vi "highlightRows.vi"(8 "error in (no error)":errorcluster, 10 "Goal.lvclass":refnum<class "Goal.lvclass">, 11 "TransactionListUserInterface in":refnum<class "TransactionListUserInterface.lvclass">) -> (0 "error out":errorcluster, 3 "TransactionListUserInterface out":refnum<class "TransactionListUserInterface.lvclass">)   [LabVIEW 2018, in "TransactionListUserInterface.lvclass"]
uses:
  TransactionListUserInterface.lvclass
  Goal/Goal.lvclass
  TransactionListUserInterface.lvclass/TransactionListUserInterface.ctl
  <vilib>/Utility/miscctls.llb/LVRowAndColumnTypeDef.ctl
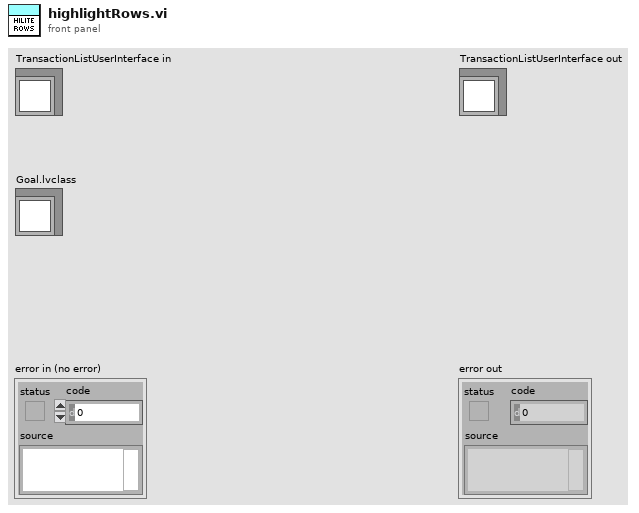
[diagram p1: front panel]
types:
  T1 = typedef "LVRowAndColumnTypeDef.ctl" = cluster{"Row":i32, "Column":i32}
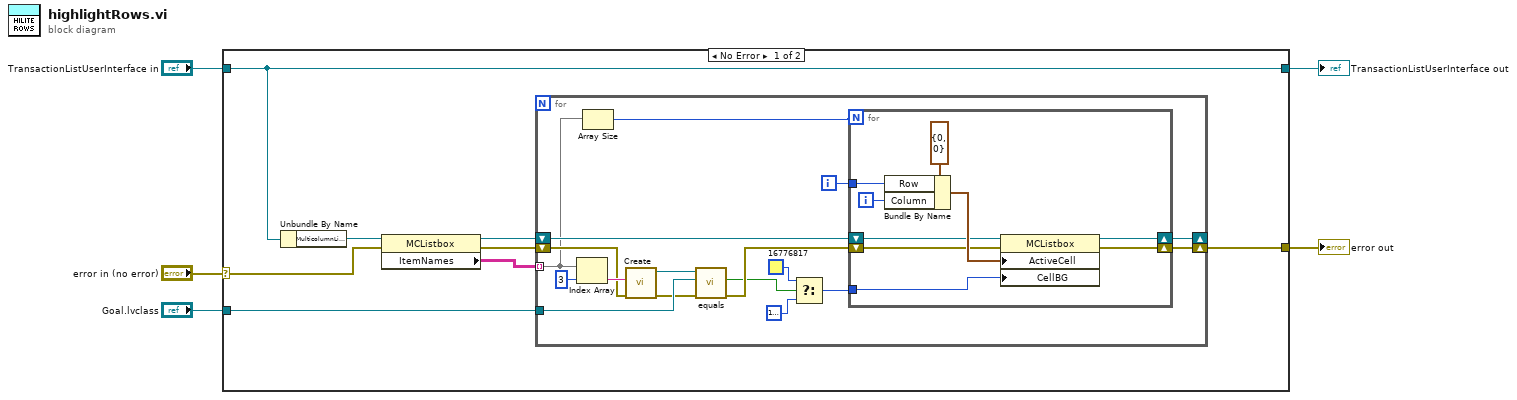
[diagram p0: block diagram]
diagram:
  n1 = case shown="No Error" "error in (no error)" {
    selector: "error in (no error)" -> [w8 w40]
    tunnel: "TransactionListUserInterface in" -> [w9 w41]
    tunnel: [w9 w41] -> w4
    tunnel: "Goal.lvclass" -> [w7 _]
    tunnel: [w6 w40] -> w1
    frame No Error {
      n2 = Unbundle By Name(w9) -> ("MulticolumnListbox"=w10:refnum<vi>)
      n3 = property on="Property Node" class="MCListbox"(reference=w10, error in=w8) -> (reference out=w12:refnum<vi>, error out=w11:errorcluster, "ItemNames"=w13:string[][])
      n4 = for {
        tunnel: w13 -> [w15] mode=indexing
        shift-right: [w23] -> w6
        shift-left: w11 -> [w19]
        shift-right: [w24] -> _
        shift-left: w12 -> [w25]
        tunnel: w7 -> [w20]
        i -> [w29]
        n5 = Index Array(array=w15, index=3) -> (element=w22:string)
        n6 = Array Size(array=w15) -> (size(s)=w14:i32)
        n7 = call "Create.vi"("error in (no error)"=w19, "Category Name"=w22) -> ("error out"=w18:errorcluster, "Goal out"=w21:refnum<class "Goal.lvclass">)  [unwired: 8 in]
        n8 = call "equals.vi"("error in (no error)"=w18, "Goal to Match"=w20, "Goal in"=w21) -> ("error out"=w17:errorcluster, "Equals?"=w16:bool)  [unwired: 6 in, 1 out]
        n9 = Select(t=u32 16776817, s=w16, f=u32 16777216) -> (s? t:f=w26:u32)
        n10 = for {
          N: w14 -> [_]
          tunnel: w29 -> [w39]
          tunnel: w26 -> [w35]
          shift-right: [w32] -> w23
          shift-left: w17 -> [w33]
          shift-right: [w31] -> w24
          shift-left: w25 -> [w34]
          i -> [w36]
          n11 = Bundle By Name(cluster=T1 {"Row"=0, "Column"=0} ("Active Cell:Active Cell"), "Row"=w39, "Column"=w36) -> (w38:T1)
          n12 = property on="Property Node" class="MCListbox"(reference=w34, error in=w33, "ActiveCell"=w38, "CellBG"=w35) -> (reference out=w31:refnum<vi>, error out=w32:errorcluster)
        }
      }
    }
    frame Error {
    }
  }
  "error out" <- w1
  "TransactionListUserInterface out" <- w4
